vi "Read Color Pair.vi"(8 "error in (no error)":errorcluster, 9 "Active Plot":i32, 11 "3D Plot in":refnum<class "3D Plot.lvclass">) -> (0 "error out":errorcluster, 2 "Color Pair Array":cluster{"Color":u32, "String":string}[](array[cluster]), 3 "3D Plot out":refnum<class "3D Plot.lvclass">)   [LabVIEW 2020, in "3D Plot.lvclass"]
uses:
  3D Plot.lvclass
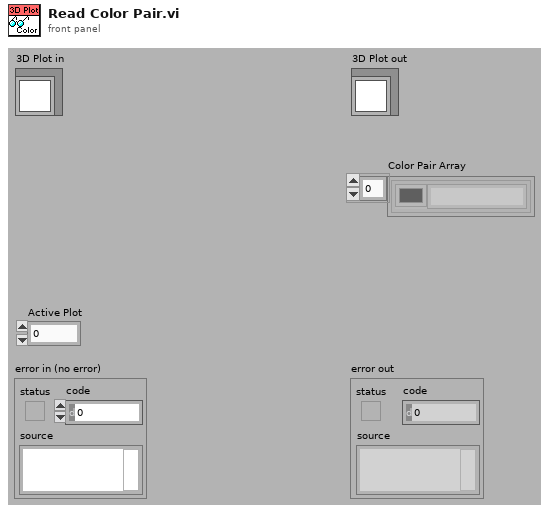
[diagram p1: front panel]
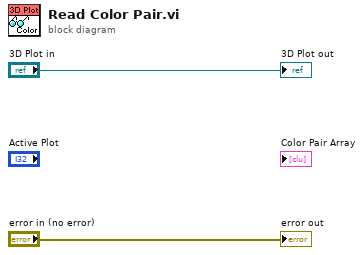
[diagram p0: block diagram]
diagram:
  "error out" <- "error in (no error)"
  "3D Plot out" <- "3D Plot in"
